vi "Read JSON.vi"(8 "error in (no error)":errorcluster, 11 "JSON Variable in":refnum<class "JSON Variable.lvclass">) -> (0 "error out":errorcluster, 2 "JSON":refnum<data-value>, 3 "JSON Variable out":refnum<class "JSON Variable.lvclass">)   [LabVIEW 2019, in "JSON Variable.lvclass"]
uses:
  JSON Variable.lvclass
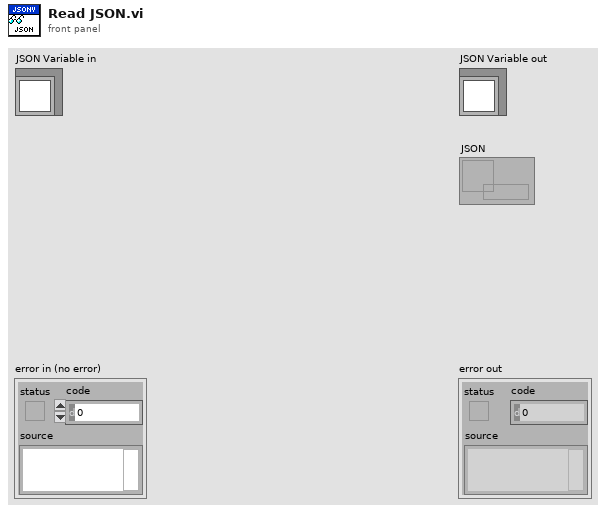
[diagram p1: front panel]
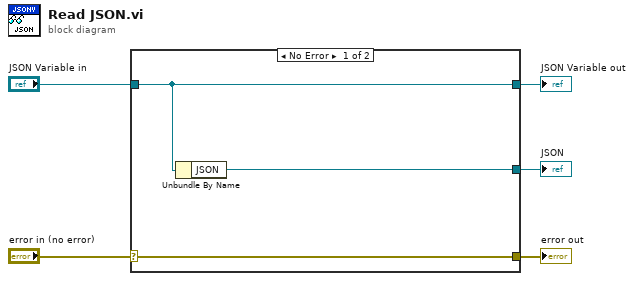
[diagram p0: block diagram]
diagram:
  n1 = case shown="No Error" "error in (no error)" {
    selector: "error in (no error)" -> [w8 w9]
    tunnel: [w8 w9] -> w4
    tunnel: [w7 w10] -> w2
    tunnel: "JSON Variable in" -> [w7 w10]
    tunnel: [w6 _] -> w1
    frame No Error {
      n2 = Unbundle By Name(w7) -> ("JSON"=w6:refnum<data-value>)
    }
    frame Error {
    }
  }
  "error out" <- w4
  "JSON Variable out" <- w2
  "JSON" <- w1
